vi "SETMODE.VI"(0 "units CONTROL DISPLAY":i8(ring) items=["K", "C", "F", "ohms"], 1 "MODE":sgl(ring) items=["LOCAL", "REMOTE", "REMOTE LL"], 2 "GPIB ADDRESS":string) -> ()   [LabVIEW 2025]
doc: "Author: Scott Hannahs <sth@magnet.fsu.edu>\n\nThis software is licensed for use under the “MIT License\"\nCopyright (c) 2025 Scott Hannahs, sth@sth@magnet.sthnet.net\n\nPermission is hereby granted, free of charge, to any person obtaining a copy of this software and associated documentation files (the \"Software\"), to deal in the Software without restriction, including without limitation the rights to use, copy, modify, merge, publish, distribute, sublicense, and/or sell copies of the Software, and to permit persons to whom the Software is furnished to do so, subject to the following conditions: The above copyright notice and this permission notice shall be included in all copies or substantial portions of the Software.\n\nTHE SOFTWARE IS PROVIDED \"AS IS\", WITHOUT WARRANTY OF ANY KIND, EXPRESS OR IMPLIED, INCLUDING BUT NOT LIMITED TO THE WARRANTIES OF MERCHANTABILITY, FITNESS FOR A PARTICULAR PURPOSE AND NONINFRINGEMENT. IN NO EVENT SHALL THE AUTHORS OR COPYRIGHT HOLDERS BE LIABLE FOR ANY CLAIM, DAMAGES OR OTHER LIABILITY, WHETHER IN AN ACTION OF CONTRACT, TORT OR OTHERWISE, ARISING FROM, OUT OF OR IN CONNECTION WITH THE SOFTWARE OR THE USE OR OTHER DEALINGS IN THE SOFTWARE."
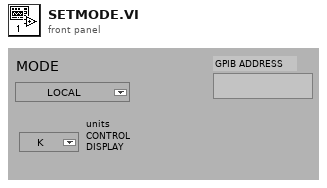
[diagram p1: front panel]
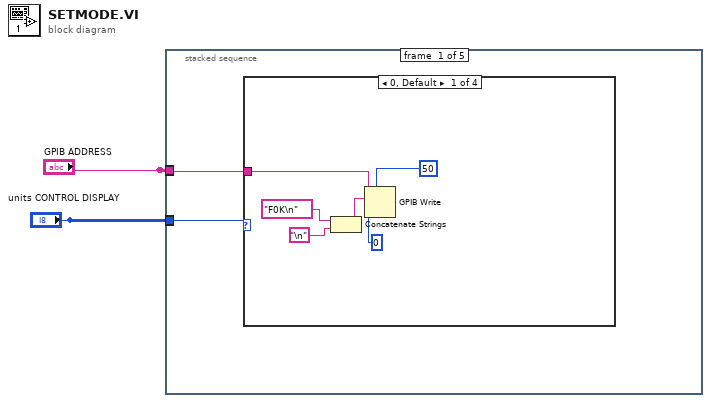
[diagram p0: block diagram]
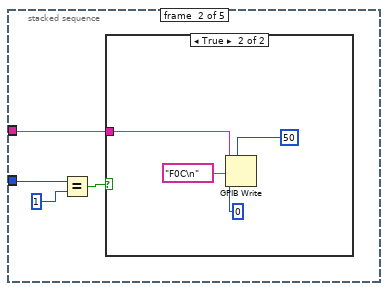
[diagram p5: hidden frame]
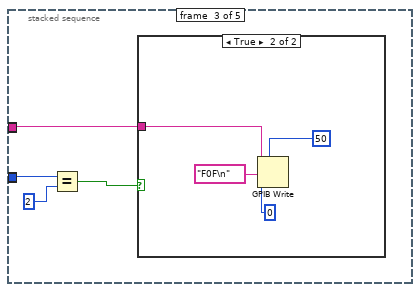
[diagram p7: hidden frame]
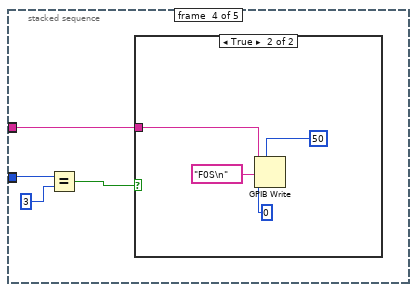
[diagram p9: hidden frame]
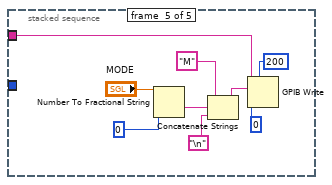
[diagram p11: hidden frame]
diagram:
  n1 = stacked-sequence {
    tunnel: "GPIB ADDRESS" -> [w4 w12 _ _ _]
    tunnel: "GPIB ADDRESS" -> [_ _ w20 _ _]
    tunnel: "GPIB ADDRESS" -> [_ _ _ w28 w40]
    tunnel: "units CONTROL DISPLAY" -> [_ w11 _ _ _]
    tunnel: "units CONTROL DISPLAY" -> [_ _ w19 w27 _]
    tunnel: "units CONTROL DISPLAY" -> [w3 _ _ _ _]
    frame #0 {
      n2 = case shown="0, Default" w3 {
        tunnel: w4 -> [w8 _ _ _]
        frame 0, Default {
          n3 = Concatenate Strings("F0K\n", "\n") -> (w7:string)
          n4 = GPIB Write(0:w8, 1:w7, 2:0, 4:50) -> ()  [unwired: 1 in, 2 out]
        }
        frame 1 {
        }
        frame 2 {
        }
        frame 3 {
        }
      }
    }
    frame #1 {
      n5 = Equal?(x=w11, y=1) -> (x = y?=w13:bool)
      n6 = case shown="True" w13 {
        tunnel: w12 -> [_ w15]
        frame False {
        }
        frame True {
          n7 = GPIB Write(0:w15, 1:"F0C\n", 2:0, 4:50) -> ()  [unwired: 1 in, 2 out]
        }
      }
    }
    frame #2 {
      n8 = Equal?(x=w19, y=2) -> (x = y?=w21:bool)
      n9 = case shown="True" w21 {
        tunnel: w20 -> [_ w23]
        frame False {
        }
        frame True {
          n10 = GPIB Write(0:w23, 1:"F0F\n", 2:0, 4:50) -> ()  [unwired: 1 in, 2 out]
        }
      }
    }
    frame #3 {
      n11 = Equal?(x=w27, y=3) -> (x = y?=w29:bool)
      n12 = case shown="True" w29 {
        tunnel: w28 -> [_ w31]
        frame False {
        }
        frame True {
          n13 = GPIB Write(0:w31, 1:"F0S\n", 2:0, 4:50) -> ()  [unwired: 1 in, 2 out]
        }
      }
    }
    frame #4 {
      n14 = Number To Fractional String(number="MODE", precision (6)=0) -> (F-format string=w35:string)  [unwired: 2 in]
      n15 = Concatenate Strings("M", w35, "\n") -> (w37:string)
      n16 = GPIB Write(0:w40, 1:w37, 2:0, 4:200) -> ()  [unwired: 1 in, 2 out]
    }
  }
